vi "transfer_lut.vi"(6 "index of element":i32, 7 "images":refnum<class "Image.lvclass">[](array[class]), 8 "error in (no error)":errorcluster, 9 "source":refnum<vi>, 10 "destination":refnum<vi>, 11 "Image in":refnum<class "Image.lvclass">) -> (0 "error out":errorcluster, 3 "Image out":refnum<class "Image.lvclass">)   [LabVIEW 2010, in "Image.lvclass"]
uses:
  Image.lvclass
  storage_mode.ctl
  ErrorController/ErrorController/class_data.vi
  ErrorController/ErrorController/ErrorController.lvclass
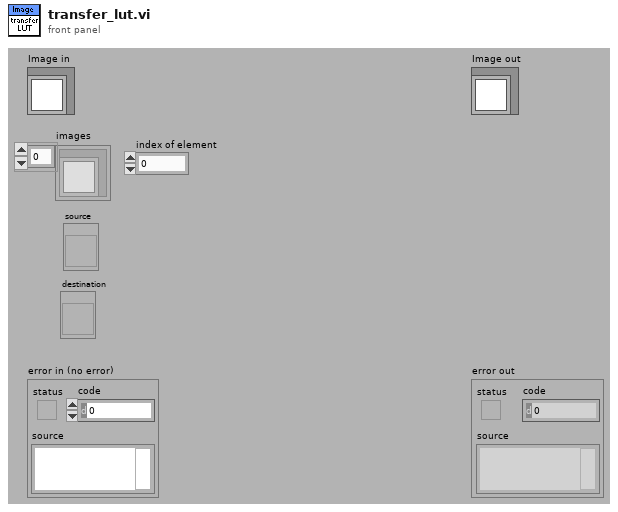
[diagram p1: front panel]
types:
  T1 = typedef "Image.lvclass/storage_mode.ctl" = enum16{"RAM", "disk"}
  T2 = typedef "IMAQ Image.ctl" = refnum<image>
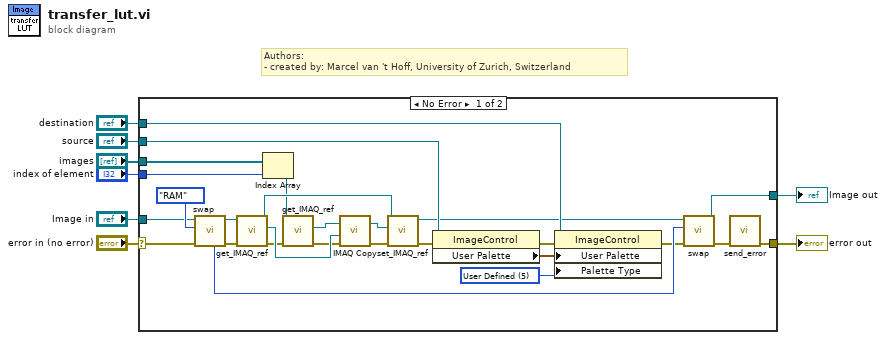
[diagram p0: block diagram]
diagram:
  # "Authors: \n- created by: Marcel van 't Hoff, University of Zurich, Switzerland"
  n1 = case shown="No Error" "error in (no error)" {
    selector: "error in (no error)" -> [w26 w37]
    tunnel: [w9 w37] -> w7
    tunnel: [w28 w36] -> w5
    tunnel: "Image in" -> [w30 w36]
    tunnel: "source" -> [w35 _]
    tunnel: "destination" -> [w33 _]
    tunnel: "images" -> [w32 _]
    tunnel: "index of element" -> [w11 _]
    frame No Error {
      w34 = u32 5 items=["Grayscale", "Binary", "Gradient", "Rainbow", "Temperature", "User Defined"] ("Palette:Palette Type")
      n2 = call-dynamic "swap.vi"("error in (no error)"=w26, "storage type target"=storage_mode."RAM", "Image in"=w30) -> ("error out"=w23:errorcluster, "Image out"=w22:refnum<class "Image.lvclass">, "previous storage mode"=w29:T1)  [unwired: 6 out]
      n3 = call-dynamic "get_IMAQ_ref.vi"("error in (no error)"=w23, "Image.lvclass in"=w22) -> ("error out"=w13:errorcluster, "Image"=w24:T2, "Image.lvclass out"=w15:refnum<class "Image.lvclass">)  [unwired: 7 out]
      n4 = Index Array(array=w32, index=w11) -> (element=w14:refnum<class "Image.lvclass">)
      n5 = call-dynamic "get_IMAQ_ref.vi"("error in (no error)"=w13, "Image.lvclass in"=w14) -> ("error out"=w12:errorcluster, "Image"=w25:T2)  [unwired: 8 out]
      n6 = call "IMAQ Copy"("error in (no error)"=w12, "Image Dst"=w24, "Image Src"=w25) -> ("error out"=w17:errorcluster, "Image Dst Out"=w16:T2)  [unwired: 3 in]
      n7 = call-dynamic "set_IMAQ_ref.vi"("error in (no error)"=w17, "Image"=w16, "Image.lvclass in"=w15) -> ("error out"=w21:errorcluster, "Image.lvclass out"=w20:refnum<class "Image.lvclass">)  [unwired: 7 in]
      n8 = property class="ImageControl"(reference=w35, error in=w21) -> (error out=w18:errorcluster, "User Palette"=w19:cluster{"Red":u8, "Green":u8, "Blue":u8}[])  [unwired: 1 out]
      n9 = property class="ImageControl"(reference=w33, error in=w18, "User Palette"=w19, "Palette Type"=w34) -> (error out=w27:errorcluster)  [unwired: 1 out]
      n10 = call-dynamic "swap.vi"("error in (no error)"=w27, "storage type target"=w29, "Image in"=w20) -> ("error out"=w10:errorcluster, "Image out"=w28:refnum<class "Image.lvclass">)  [unwired: 7 out]
      n11 = call "send_error.vi"("error in (no error)"=w10) -> ("error out"=w9:errorcluster)  [unwired: 10 in]
    }
    frame Error {
    }
  }
  "error out" <- w7
  "Image out" <- w5
